vi "PV ActiveLine - SetDegas (TPG361).vi"(7 "W/R":bool, 8 "Fehler (Eingang)":errorcluster, 10 "Gauge CH 1":i32(ring) items=["Degas off", "Degas on"], 11 "Referenz in":refnum<visa-resource-name>) -> (0 "Cluster (Ausgang)":errorcluster, 2 "Gauge CH 1 out":i32(ring) items=["Degas off", "Degas on"], 3 "Referenz out":refnum<visa-resource-name>)   [LabVIEW 2013, in "PV ActiveLine.lvlib"]
doc: "DGS - Degas\n\nDGS [,a,b]\n\nDegas gauge 1,\na =\n0 –> Degas off (default)\n1 –> Degas on (3 minutes)\n\nDegas gauge 2,\nb =\n0 –> Degas off (default)\n1 –> Degas on (3 minutes)"
uses:
  <instrlib>/PV ActiveLine/PV ActiveLine.lvlib
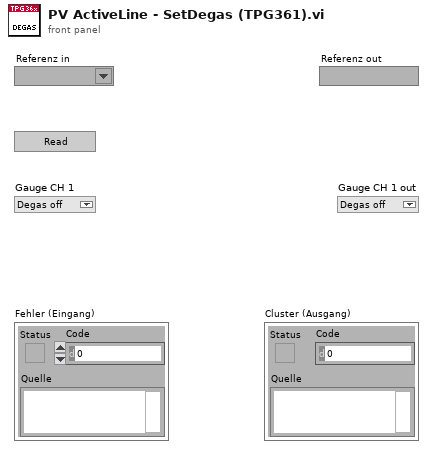
[diagram p1: front panel]
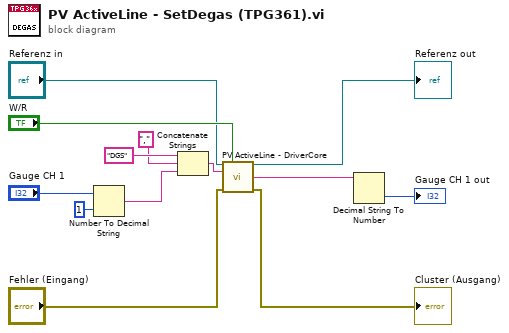
[diagram p0: block diagram]
diagram:
  n1 = Number To Decimal String(number="Gauge CH 1", width (-)=i16 1) -> (decimal integer string=w9:string)
  n2 = Concatenate Strings("DGS" ("Command"), "," ("Command"), w9) -> (w6:string)
  n3 = call <instrlib>:"PV ActiveLine - DriverCore.vi"("Referenz in"="Referenz in", "Write/Read"="W/R", "Command"=w6, "Fehler (Eingang)"="Fehler (Eingang)") -> ("Referenz out"=→"Referenz out":refnum<visa-resource-name>, "String Out"=w1:string, "Cluster (Ausgang)"=→"Cluster (Ausgang)":errorcluster)  [unwired: 9 in]
  n4 = Decimal String To Number(string=w1) -> (number=→"Gauge CH 1 out":i32)  [unwired: 2 in, 1 out]
